vi "System-Level Module.vi"() -> ()   [LabVIEW 2017]
uses:
  user.lib/_NEVSTOP/Communicable State Machine(CSM)/_Support/Priority Queue/Priority Queue.lvclass/Priority Queue.ctl
  user.lib/_NEVSTOP/Communicable State Machine(CSM)/_Support/Process/CSMP-Sync Call.vi
  user.lib/_NEVSTOP/Communicable State Machine(CSM)/Utility/uuid.vi
  user.lib/_NEVSTOP/Communicable State Machine(CSM)/Utility/Build Error Cluster.vi
  user.lib/_NEVSTOP/Communicable State Machine(CSM)/Utility/Trim Both Whitespace.vi
  user.lib/_NEVSTOP/Communicable State Machine(CSM)/_Support/CSMQ/_CSMObj-Message Check.vi
  user.lib/_NEVSTOP/Communicable State Machine(CSM)/_Support/CSMQ/_CSMObj-Enqueue Cross-Module Message.vi
  user.lib/_NEVSTOP/Communicable State Machine(CSM)/_Support/CSMQ/_CSMOFGV Get.vi
  user.lib/_NEVSTOP/Communicable State Machine(CSM)/_Support/Priority Queue/Enqueue Element.vi
  user.lib/_NEVSTOP/Communicable State Machine(CSM)/_Support/FGV-BroadcastRegistry/global-CSMQ FGV Change Flag.vi
  user.lib/_NEVSTOP/Communicable State Machine(CSM)/_Support/CSMQ/_CSMOFGV.vi
  user.lib/_NEVSTOP/Communicable State Machine(CSM)/_Support/Error/CSM No Target Error.vi
  user.lib/_NEVSTOP/Communicable State Machine(CSM)/_Support/Error/CSM Not Allowed Message.vi
  user.lib/_NEVSTOP/Communicable State Machine(CSM)/_Support/Error/CSM Target Error.vi
  user.lib/_NEVSTOP/Communicable State Machine(CSM)/_Support/Error/CSM Unhandled State Error.vi
  user.lib/_NEVSTOP/Communicable State Machine(CSM)/_Support/Error/CSM Target Timeout Error.vi
  user.lib/_NEVSTOP/Communicable State Machine(CSM)/Communicable State Machine.lvlib
panel:
  out "Module Names":string[](array[string])
  out "error out":errorcluster
  out "CSM Name(marked as Sysetem-Level Module)":string
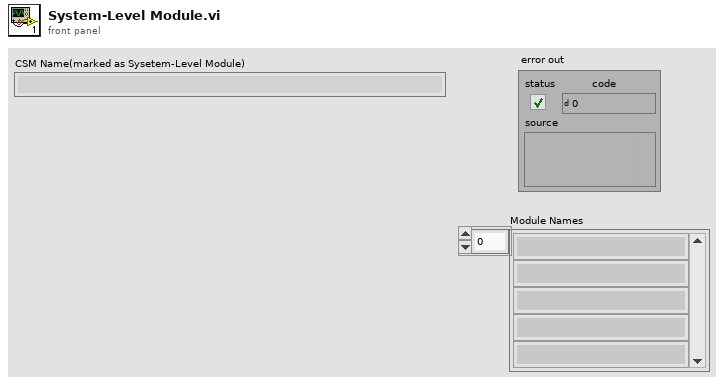
[diagram p1: front panel]
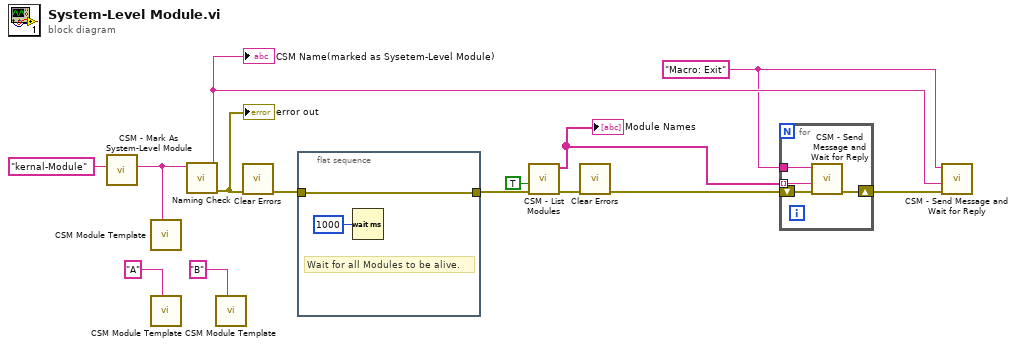
[diagram p0: block diagram]
diagram:
  w2 = "Macro: Exit" ("CSM Name")
  n1 = call "CSM - Mark As System-Level Module.vi"("CSM Name"="kernal-Module") -> ("CSM Name(marked as Sysetem-Level Module)"=w13:string)  [unwired: 9 in]
  n2 = call "CSM Module Template.vi"("Name(\"\" to use uuid)"=w13) -> ()  [unwired: 11 in]
  n3 = call "CSM Module Template.vi"("Name(\"\" to use uuid)"="A" ("Name(\"\" to use uuid)")) -> ()  [unwired: 11 in]
  n4 = call "Naming Check.vi"("Name(\"\" to use uuid)"=w13) -> ("error out"=w12:errorcluster, "Name(dup)"=w8:string)  [unwired: 9 in]
  "CSM Name(marked as Sysetem-Level Module)" <- w8
  "error out" <- w12
  n5 = call "CSM Module Template.vi"("Name(\"\" to use uuid)"="B" ("Name(\"\" to use uuid)")) -> ()  [unwired: 11 in]
  n6 = call <vilib>:"Clear Errors.vi"("error in (no error)"=w12) -> ("error out"=w10:errorcluster)  [unwired: 5 in, 1 out]
  n7 = flat-sequence {
    tunnel: [w15] -> w11
    tunnel: w10 -> [w15]
    frame #0 {
      # "Wait for all Modules to be alive."
      n8 = Wait (ms)(milliseconds to wait=u32 1000) -> ()  [unwired: 1 out]
    }
  }
  n9 = call "CSM - List Modules.vi"("Error in"=w11, "All?"=TRUE) -> ("Error out"=w9:errorcluster, "Module Names"=w1:string[])  [unwired: 8 in]
  "Module Names" <- w1
  n10 = call <vilib>:"Clear Errors.vi"("error in (no error)"=w9) -> ("error out"=w6:errorcluster)  [unwired: 5 in, 1 out]
  n11 = for {
    tunnel: w2 -> [w18]
    shift-right: [w19] -> w5
    shift-left: w6 -> [w20]
    tunnel: w1 -> [w17] mode=indexing
    n12 = call "CSM - Send Message and Wait for Reply.vi"("Error In (no error)"=w20, "Target Module"=w17, "State"=w18) -> ("error out"=w19:errorcluster)  [unwired: 6 in, 2 out]
  }
  n13 = call "CSM - Send Message and Wait for Reply.vi"("Error In (no error)"=w5, "Target Module"=w8, "State"=w2) -> ()  [unwired: 6 in, 3 out]
